vi "Validate Hardware.vi"(6 "Interactive":bool, 8 "error in (no error)":errorcluster, 9 "Pane":refnum<vi>, 10 "XY graph ref":refnum<vi>, 11 "Spectrum Recorder in":refnum<class "Spectrum Recorder.lvclass">) -> (0 "error out":errorcluster, 2 "Valid":bool, 3 "Spectrum Recorder out":refnum<class "Spectrum Recorder.lvclass">)   [LabVIEW 2016, in "Spectrum Recorder.lvclass"]
uses:
  Spectrum Recorder.lvclass
  Utilities/Cursor Digitizer/Cursor Digitizer.lvclass
  C:/Program Files/National Instruments/LabVIEW 2016/vi.lib/ActorFramework/Actor/Actor.lvclass
  Spectrum Recorder.lvclass/Spectrum Recorder.ctl
  Utilities/Cursor Digitizer/Cursor Digitizer.lvclass/Cursor Digitizer.ctl
  Utilities/Cursor Digitizer/Write XY graph ref.vi
  Utilities/Cursor Digitizer/Write Callers pane.vi
  Red Pitaya/RP Core/RP Transceiver/RP Transceiver.lvclass
  <vilib>/ActorFramework/Actor/Actor.lvclass
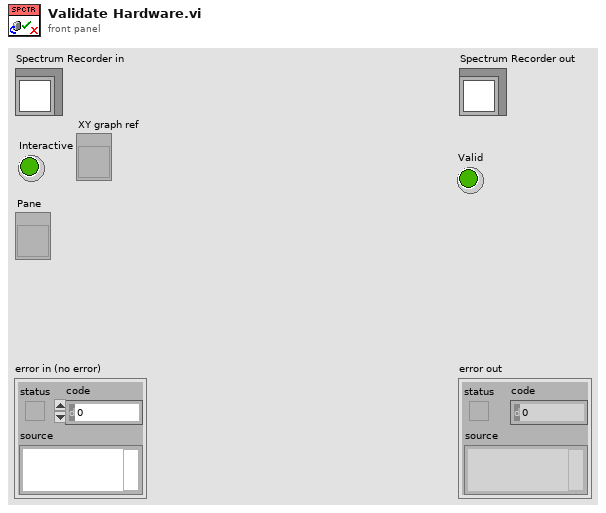
[diagram p1: front panel]
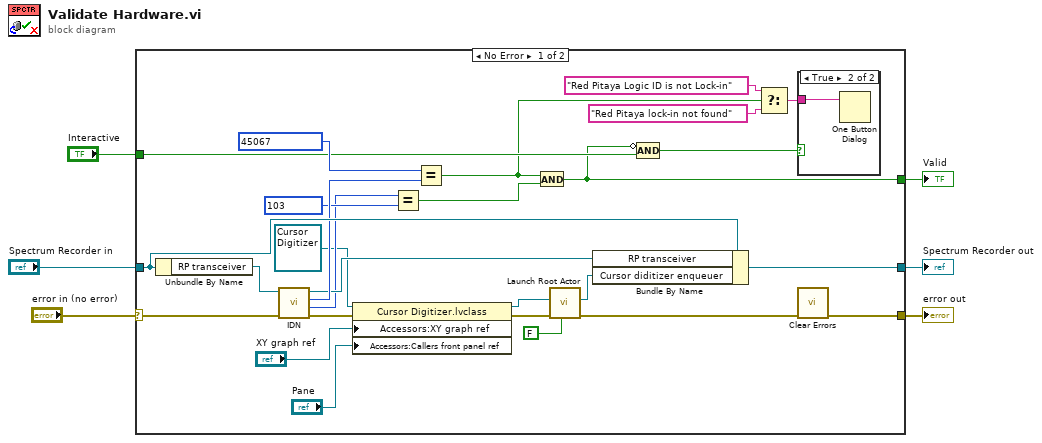
[diagram p0: block diagram]
diagram:
  n1 = case shown="No Error" "error in (no error)" {
    selector: "error in (no error)" -> [w29 w36]
    tunnel: [w21 w36] -> w5
    tunnel: [w28 w35] -> w3
    tunnel: "Spectrum Recorder in" -> [w33 w35]
    tunnel: [w22 _] -> w2
    tunnel: "Interactive" -> [w23 _]
    frame No Error {
      n2 = Unbundle By Name(w33) -> ("RP transceiver"=w32:refnum<class "RP Transceiver.lvclass">)
      n3 = call-dynamic "IDN.vi"("error in (no error)"=w29, "RP Instrument in"=w32) -> ("error out"=w15:errorcluster, "Logic tag"=w25:u16, "IDN response"=w30:u32, "RP Instrument out"=w27:refnum<class "RP Transceiver.lvclass">)  [unwired: 6 in]
      n4 = property class="Cursor Digitizer.lvclass"(reference=refnum<class "Cursor Digitizer.lvclass"> refnum ("Cursor Digitizer.lvclass"), error in=w15, "Accessors:XY graph ref"="XY graph ref", "Accessors:Callers front panel ref"="Pane") -> (reference out=w9:refnum<class "Cursor Digitizer.lvclass">, error out=w11:errorcluster)
      n5 = Equal?(x=w25, y=u16 103 ("IDN response")) -> (x = y?=w24:bool)
      n6 = Equal?(x=u32 45067 ("IDN response"), y=w30) -> (x = y?=w19:bool)
      n7 = And(x=w19, y=w24) -> (x .and. y?=w22:bool)
      n8 = call <vilib>:"Launch Root Actor.vi"("Open Actor Core front panel? (F)"=FALSE, "error in (no error)"=w11, "Actor"=w9) -> ("error out"=w14:errorcluster, "Actor's Enqueuer"=w12:refnum<class "Message Enqueuer.lvclass">)  [unwired: 7 in]
      n9 = Bundle By Name(cluster=w33, "RP transceiver"=w27, "Cursor diditizer enqueuer"=w12) -> (w28:refnum<class "Spectrum Recorder.lvclass">)
      n10 = Compound Arithmetic op=AND(invert w22, w23) -> (w20:bool)
      n11 = Select(t="Red Pitaya Logic ID is not Lock-in" ("message"), s=w19, f="Red Pitaya lock-in not found" ("message")) -> (s? t:f=w16:string)
      n12 = case shown="True" w20 {
        tunnel: w16 -> [_ w34]
        frame False {
        }
        frame True {
          n13 = One Button Dialog(message=w34) -> ()  [unwired: 1 in, 1 out]
        }
      }
      n14 = call <vilib>:"Clear Errors.vi"("error in (no error)"=w14) -> ("error out"=w21:errorcluster)  [unwired: 5 in, 1 out]
    }
    frame Error {
    }
  }
  "error out" <- w5
  "Spectrum Recorder out" <- w3
  "Valid" <- w2
